vi "Decode Scan Data.vi"(8 "error in (no error)":errorcluster, 10 "Data":string, 11 "Packet in":refnum<class "Packet.lvclass">) -> (0 "error out":errorcluster, 3 "Packet out":refnum<class "Packet.lvclass">)   [LabVIEW 2019, in "Packet.lvclass"]
uses:
  Packet.lvclass
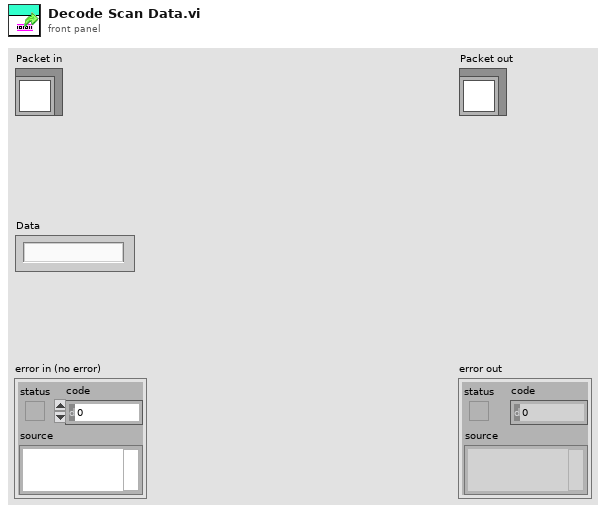
[diagram p1: front panel]
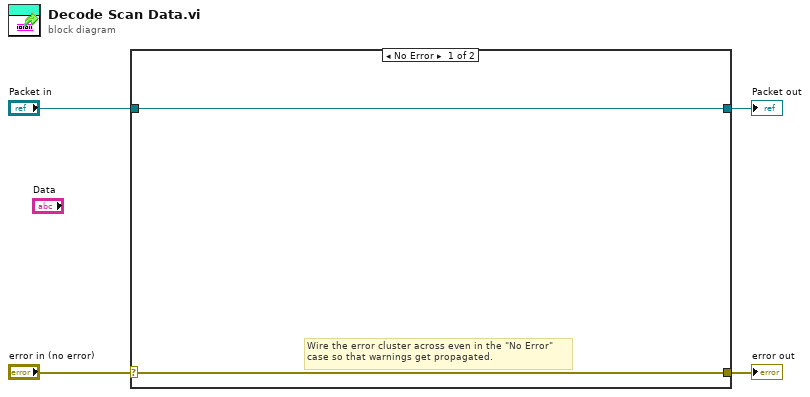
[diagram p0: block diagram]
diagram:
  n1 = case shown="No Error" "error in (no error)" {
    selector: "error in (no error)" -> [w5 w8]
    tunnel: [w5 w8] -> w3
    tunnel: [w6 w7] -> w1
    tunnel: "Packet in" -> [w6 w7]
    frame No Error {
      # "Wire the error cluster across even in the \"No Error\"\ncase so that warnings get propagated."
    }
    frame Error {
    }
  }
  "error out" <- w3
  "Packet out" <- w1
